vi "queue_state_&_argument (Single).vi"(6 "Priority? (F)":bool, 8 "error in (no error)":errorcluster, 10 "state:argument":string, 11 "Queue in":refnum<queue>) -> (0 "error out":errorcluster, 3 "Queue out":refnum<queue>)   [LabVIEW 2015]
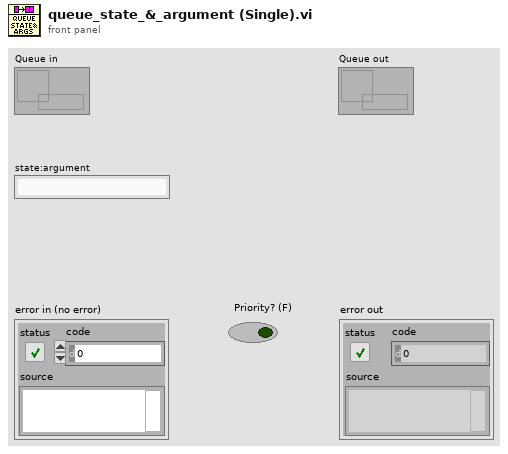
[diagram p1: front panel]
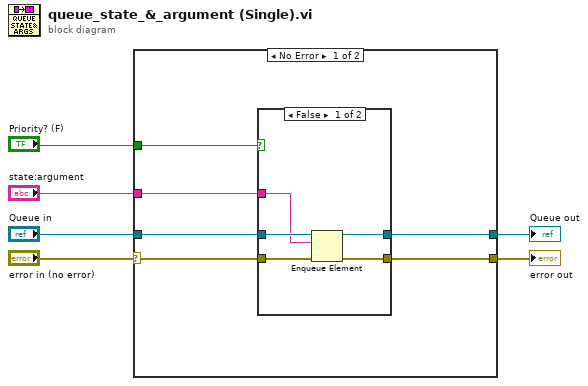
[diagram p0: block diagram]
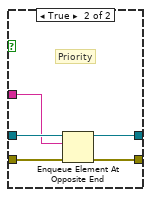
[diagram p2: hidden frame]
diagram:
  n1 = case shown="No Error" "error in (no error)" {
    selector: "error in (no error)" -> [w12 w24]
    tunnel: [w11 w24] -> w3
    tunnel: "state:argument" -> [w7 _]
    tunnel: "Queue in" -> [w10 w23]
    tunnel: [w9 w23] -> w6
    tunnel: "Priority? (F)" -> [w8 _]
    frame No Error {
      n2 = case shown="False" w8 {
        tunnel: w12 -> [w17 w22]
        tunnel: w10 -> [w16 w20]
        tunnel: [w15 w19] -> w9
        tunnel: w7 -> [w14 w18]
        tunnel: [w13 w21] -> w11
        frame False {
          n3 = Enqueue Element(queue=w16, element=w14, error in (no error)=w17) -> (queue out=w15:refnum<queue>, error out=w13:errorcluster)  [unwired: 1 in, 1 out]
        }
        frame True {
          # "Priority"
          n4 = Enqueue Element At Opposite End(queue=w20, element=w18, error in (no error)=w22) -> (queue out=w19:refnum<queue>, error out=w21:errorcluster)  [unwired: 1 in, 1 out]
        }
      }
    }
    frame Error {
    }
  }
  "error out" <- w3
  "Queue out" <- w6
